vi "IndColor.vi"(10 "Warning":bool) -> (2 "IndColor":cluster{"BGColor":dbl, "TextColor":dbl})   [LabVIEW 2016]
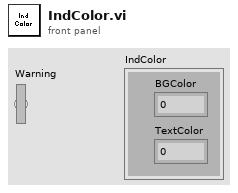
[diagram p1: front panel]
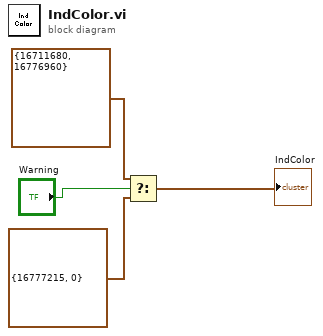
[diagram p0: block diagram]
diagram:
  n1 = Select(t=cluster{i32, i32} {16711680, 16776960}, s="Warning", f=cluster{i32, i32} {16777215, 0}) -> (s? t:f=→"IndColor":cluster{i32, i32})
